vi "containing bix.vi"(11 "z in":cdb[](array[numeric])) -> (2 "norm":dbl, 3 "center":cdb)   [LabVIEW 2018]
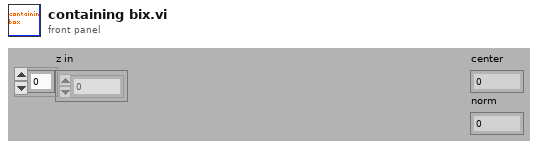
[diagram p1: front panel]
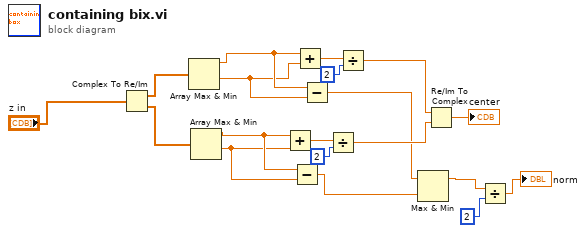
[diagram p0: block diagram]
diagram:
  n1 = Complex To Re/Im(x + iy="z in") -> (x=w18:dbl[], y=w17:dbl[])
  n2 = Array Max & Min(array=w18) -> (max value=w16:dbl, min value=w9:dbl)  [unwired: 2 out]
  n3 = Array Max & Min(array=w17) -> (max value=w11:dbl, min value=w10:dbl)  [unwired: 2 out]
  n4 = Add(x=w11, y=w10) -> (x+y=w13:dbl)
  n5 = Subtract(x=w11, y=w10) -> (x-y=w4:dbl)
  n6 = Add(x=w16, y=w9) -> (x+y=w15:dbl)
  n7 = Subtract(x=w16, y=w9) -> (x-y=w5:dbl)
  n8 = Divide(x=w13, y=2) -> (x/y=w7:dbl)
  n9 = Divide(x=w15, y=2) -> (x/y=w8:dbl)
  n10 = Max & Min(x=w5, y=w4) -> (max(x,y)=w2:dbl)  [unwired: 1 out]
  n11 = Re/Im To Complex(1:w7, 2:w8) -> (0:→"center":cdb)
  n12 = Divide(x=w2, y=2) -> (x/y=→"norm":dbl)
